vi "MHX Tube Measurements.vi"(9 "MHX Tube Diameter":dbl, 10 "MHX Length":dbl, 11 "MHX Tube Wall Thickness":dbl) -> (1 "Am (m^2)":dbl, 2 "Ai (m^2)":dbl, 3 "Ao (m^2)":dbl)   [LabVIEW 2019]
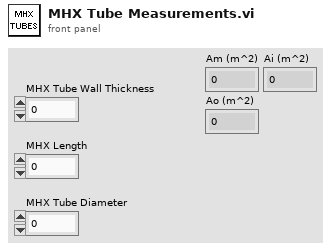
[diagram p1: front panel]
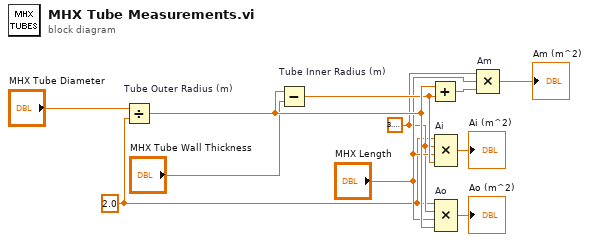
[diagram p0: block diagram]
diagram:
  w7 = 3.141592653589793
  w6 = 2.0 ("y")
  n1 = Divide "Tube Outer Radius (m)"(x="MHX Tube Diameter", y=w6) -> (x/y=w11:dbl)
  n2 = Subtract "Tube Inner Radius (m)"(x=w11, y="MHX Tube Wall Thickness") -> (x-y=w10:dbl)
  n3 = Add(x=w11, y=w10) -> (x+y=w9:dbl)
  n4 = Compound Arithmetic op=MULTIPLY "Ai"(w6, w7, "MHX Length", w10) -> (→"Ai (m^2)":dbl)
  n5 = Compound Arithmetic op=MULTIPLY "Ao"(w6, w7, "MHX Length", w11) -> (→"Ao (m^2)":dbl)
  n6 = Compound Arithmetic op=MULTIPLY "Am"(w7, "MHX Length", w9) -> (→"Am (m^2)":dbl)
